vi "All Child Values.vi"(11 "NewEntityTemplate in":refnum<class "NewEntityTemplate.lvclass">) -> (2 "All Values":refnum<class "Type.lvclass">[](array[class]))   [LabVIEW 2020, in "NewEntityTemplate.lvclass"]
uses:
  NewEntityTemplate.lvclass
  Conditum/Columns/Type/Type.lvclass
  NewEntityTemplate.lvclass/NewEntityTemplate.ctl
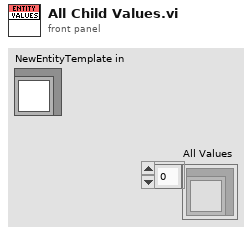
[diagram p1: front panel]
types:
  T1 = typedef "NewEntityTemplate.lvclass/Columns.ctl" = cluster{"Placeholder":refnum<class "Type.lvclass">}
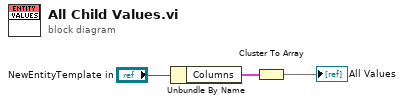
[diagram p0: block diagram]
diagram:
  n1 = Unbundle By Name("NewEntityTemplate in") -> ("Columns"=w2:T1)
  n2 = Cluster To Array(cluster=w2) -> (array=→"All Values":refnum<class "Type.lvclass">[])
